vi "Overwrite-all-hidden-params.vi"(8 "error in (no error)":errorcluster, 10 "Storage params adv":T1={"Storage labels"={"Original"="Original", "Corrected"="Corrected", "Binary"="Binary", "Temperature"="Temperature", "Characteristics"="Characteristics", "Mapping"="Mapping", "TemperatureValues"="TemperatureValues"}, "Characteristics headers"=["Average intensity [0-255]", "Peak intensity [0-255]", "Melt-pool size [mm²]", "Melt-pool aspect ratio []", "Melt-pool fragments []"], "CharacteristicsTemperature headers"=["Melt-pool center X [pixel]", "Melt-pool center Y [pixel]", "Orientation []"]}, 11 "Storage params. ref. in":refnum<data-value>) -> (0 "error out":errorcluster, 3 "Storage params. ref.":refnum<data-value>)   [LabVIEW 2013, in "CameraVision.lvlib" / "CV-Storage.lvclass"]
uses:
  CV-Storage.lvclass
  Storage-parameters-advanced.ctl
  Storage-types-labels.ctl
  CV-Storage.lvclass/CV-Storage.ctl
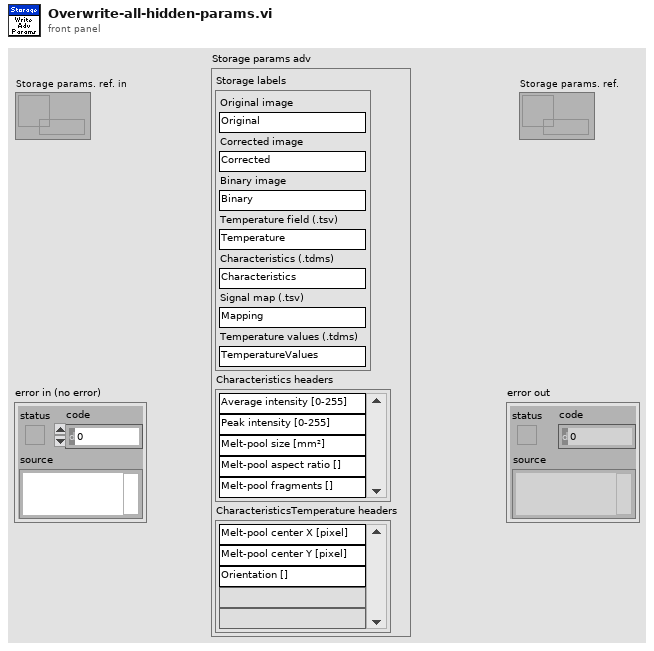
[diagram p1: front panel]
types:
  T1 = typedef "CameraVision.lvlib/CV-Storage.lvclass/Storage-parameters-advanced.ctl" = cluster{"Storage labels":T2, "Characteristics headers":string[], "CharacteristicsTemperature headers":string[]}
  T2 = typedef "CameraVision.lvlib/CV-Storage.lvclass/Storage-types-labels.ctl" = cluster{"Original":string, "Corrected":string, "Binary":string, "Temperature":string, "Characteristics":string, "Mapping":string, "TemperatureValues":string}
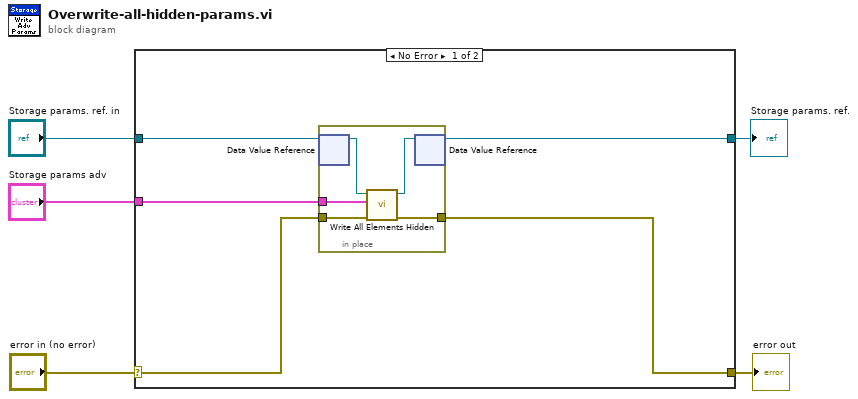
[diagram p0: block diagram]
diagram:
  n1 = case shown="No Error" "error in (no error)" {
    selector: "error in (no error)" -> [w8 w17]
    tunnel: [w9 w17] -> w4
    tunnel: "Storage params. ref. in" -> [w7 w16]
    tunnel: "Storage params adv" -> [w10 _]
    tunnel: [w6 w16] -> w1
    frame No Error {
      n2 = in-place {
        in-place-border: w10 -> [w13]
        in-place-border: [w11] -> w9
        in-place-border: w8 -> [w12]
        n3 = in-place-dvr #1(w7) -> (w14:refnum<class "CV-Storage.lvclass">)  [unwired: 1 out]
        n4 = call "Write All Elements Hidden.vi"("error in (no error)"=w12, "Storage params. hidden"=w13, "Storage params in"=w14) -> ("error out"=w11:errorcluster, "Storage params out"=w15:refnum<class "CV-Storage.lvclass">)  [unwired: 7 in]
        n5 = in-place-dvr #1(w15) -> (w6:refnum<data-value>)  [unwired: 1 out]
      }
    }
    frame Error {
    }
  }
  "error out" <- w4
  "Storage params. ref." <- w1
